vi "Equi-Ripple HighPass PtByPt.vi"(4 "initialize":bool, 5 "stop freq":dbl=0.2 format="%0.2f", 6 "high freq":dbl=0.25 format="%0.2f", 7 "# of taps":i32=31, 9 "sampling freq: fs":dbl=1.0 format="%0.2f", 10 "x":dbl format="%0.2f") -> (0 "error":i32, 3 "Filtered x":dbl format="%0.2f")   [LabVIEW 2020, in "NI_PtbyPt.lvlib"]
doc: "Filters <B>x</B> using an equi-ripple highpass FIR filter model."
uses:
  NI_PtbyPt.lvlib
  NI_AALBase.lvlib
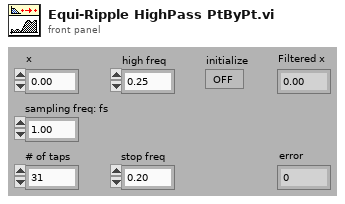
[diagram p1: front panel]
types:
  T1 = cluster{"Amplitude":dbl, "DC":dbl, "stop freq":dbl, "Weight":dbl}
  T2 = cluster{"Amplitude":dbl, "high freq":dbl, dbl, "Weight":dbl}
  T3 = cluster{"Amplitude":dbl, "high freq":dbl, "stop freq":dbl, "Weight":dbl}[]
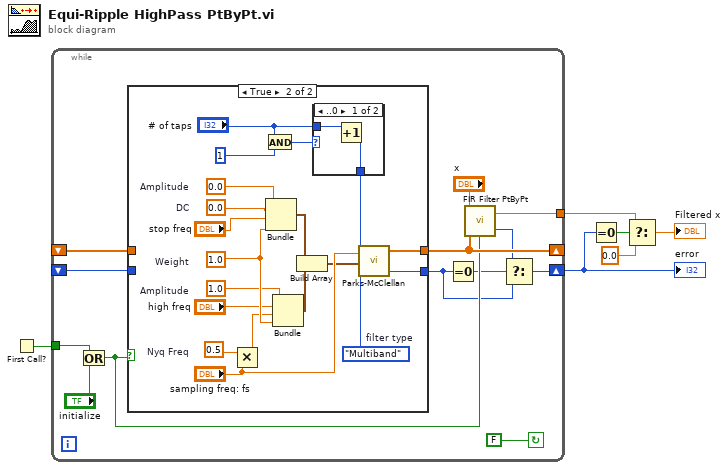
[diagram p0: block diagram]
diagram:
  n1 = First Call?() -> (First Call?: T/F=w6:bool)
  n2 = while {
    tunnel: w6 -> [w15]
    shift-left: _ -> [w17]
    shift-right: [w19] -> _
    shift-right: [w9] -> w5
    shift-left: _ -> [w8]
    tunnel: [w7] -> w3
    stop <- FALSE continue-if-true
    n3 = Or(x=w15, y="initialize") -> (x .or. y?=w13:bool)
    n4 = case shown="True" w13 {
      tunnel: [w21 w40] -> w19
      tunnel: w17 -> [w21 _]
      tunnel: [w20 w22] -> w10
      tunnel: w8 -> [w20 _]
      frame False {
      }
      frame True {
        w38 = 0.0  # Amplitude
        w39 = 0.0  # DC
        w36 = 1.0  # Amplitude
        w25 = 0.5  # Nyq Freq
        w37 = 1.0  # Weight
        w33 = enum32{"Multiband", "Differentiator", "Hilbert"}."Multiband"  # filter type
        n5 = Multiply(x=w25, y="sampling freq: fs") -> (x*y=w26:dbl)
        n6 = And(x="# of taps", y=1) -> (x .and. y?=w30:i32)
        n7 = Bundle("Amplitude"=w38, "DC"=w39, "stop freq"="stop freq", "Weight"=w37) -> (w27:T1)  [unwired: 1 out]
        n8 = Bundle("Amplitude"=w36, "high freq"="high freq", w26, "Weight"=w37) -> (w28:T2)  [unwired: 1 out]
        n9 = Build Array(w27, w28) -> (w34:T3)
        n10 = case shown="..0" w30 {
          tunnel: "# of taps" -> [w42 w43]
          tunnel: [w41 w43] -> w32
          frame ..0 {
            n11 = Increment(x=w42) -> (x+1=w41:i32)
          }
          frame 1.. {
          }
        }
        n12 = call "Parks-McClellan.vi"("filter type"=w33, "Band Parameters"=w34, "sampling freq: fs"="sampling freq: fs", "# of taps"=w32) -> ("error"=w22:i32, "h"=w40:dbl[])  [unwired: 1 out]
      }
    }
    n13 = Equal To 0?(x=w10) -> (x = 0?=w12:bool)
    n14 = call "FIR Filter PtByPt.vi"("initialize"=w13, "Forward Coefficients"=w19, "x"="x") -> ("error"=w11:i32, "Filtered x"=w7:dbl)  [unwired: 1 out]
    n15 = Select(t=w11, s=w12, f=w10) -> (s? t:f=w9:i32)
  }
  "error" <- w5
  n16 = Equal To 0?(x=w5) -> (x = 0?=w4:bool)
  n17 = Select(t=w3, s=w4, f=0.0) -> (s? t:f=→"Filtered x":dbl)
